vi "Get File Extension and Name Without Extension.vi"(11 "file":path) -> (2 "lowercase file extension":string, 3 "filename without extension":string)   [LabVIEW 2015]
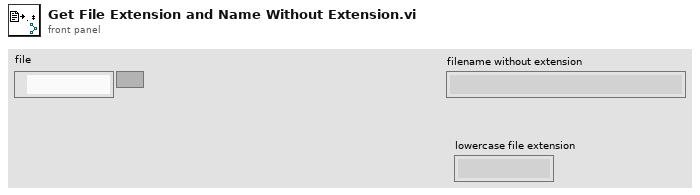
[diagram p1: front panel]
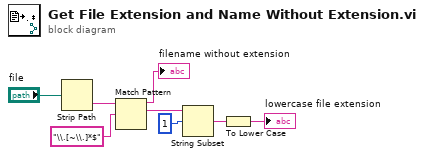
[diagram p0: block diagram]
diagram:
  n1 = Strip Path(path="file") -> (name=w7:string)  [unwired: 1 out]
  n2 = Match Pattern(string=w7, regular expression="\\.[~\\.]*$") -> (before substring=→"filename without extension":string, match substring=w4:string)  [unwired: 1 in, 2 out]
  n3 = String Subset(string=w4, offset (0)=1) -> (substring=w2:string)  [unwired: 1 in]
  n4 = To Lower Case(string=w2) -> (all lower case string=→"lowercase file extension":string)
